vi "ActionVIOnDelete_RemoveSystemMappings.vi"(6 "All deleted Refs":T1[](array[typedef]) format="%.0x", 8 "error in (no error)":errorcluster, 11 "Item Ref in":T1 format="%.0x") -> (0 "error out":errorcluster, 3 "Item Ref out":T1 format="%.0x")   [LabVIEW 2015, in "Protection and Rolling Counter Addon System Explorer.lvlib"]
uses:
  Protection and Rolling Counter Addon System Explorer.lvlib
  <vilib>/NI Veristand/Custom Device API/Custom Device Item Ref.ctl
  Shared/Protection and Rolling Counter Addon Shared.lvlib
  <vilib>/NI Veristand/Custom Device API/Custom Device API.lvlib
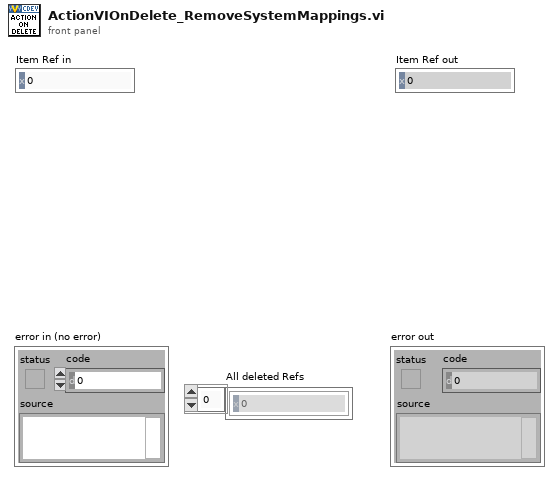
[diagram p1: front panel]
types:
  T1 = typedef "Custom Device API.lvlib/Custom Device Item Ref.ctl" = u64
  T2 = typedef "Protection and Rolling Counter Addon Shared.lvlib/FrameConfiguration.ctl" = cluster{"Input Channels":T3[], "Frame Rate":dbl, "Rolling Counter Count":dbl, "PCL Count":u64, "Max Count":dbl, "Frame ID":u32, "Rolling Counter":T3, "CRC":T3, "Frame Name":string, "Cluster":string, "Database":string, "Protection Type":T4}
  T3 = typedef "Protection and Rolling Counter Addon Shared.lvlib/InputChannelConfiguration.ctl" = cluster{"Start Bit":i32, "Name":string, "Node Path":string, "Number of bits":i32, "Scale":dbl, "Offset":dbl, "Data Type":u32}
  T4 = typedef "Protection and Rolling Counter Addon Shared.lvlib/Protection Type.ctl" = enum16{"Checksum", "CRC", "None (Counter Only)"}
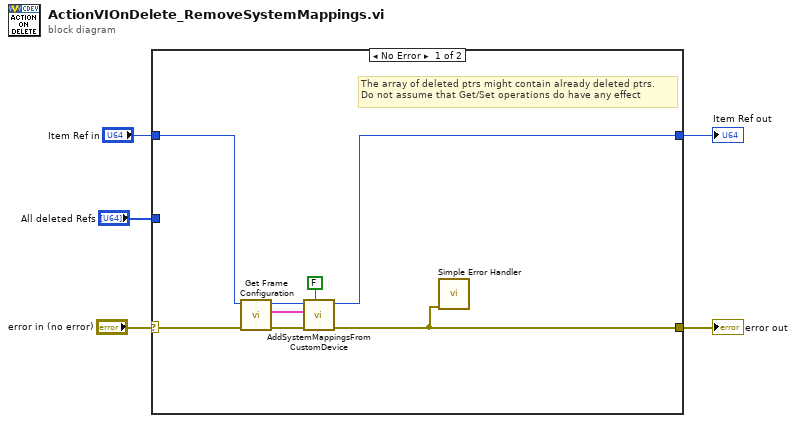
[diagram p0: block diagram]
diagram:
  n1 = case shown="No Error" "error in (no error)" {
    selector: "error in (no error)" -> [w12 w15]
    tunnel: [w6 w15] -> w4
    tunnel: "Item Ref in" -> [w11 w14]
    tunnel: [w8 w14] -> w2
    tunnel: "All deleted Refs" -> [_ _]
    frame No Error {
      # "The array of deleted ptrs might contain already deleted ptrs.\nDo not assume that Get/Set operations do have any effect"
      n2 = call "Get Frame Configuration.vi"("error in"=w12, "Parent Ref"=w11) -> ("error out"=w7:errorcluster, "Selected Channels"=w10:T2, "Parent Ref Out"=w9:T1)  [unwired: 7 in]
      n3 = call "AddSystemMappingsFromCustomDevice.vi"("Add? (T)"=FALSE, "error in"=w7, "Frame Configuration"=w10, "Node Ptr"=w9) -> ("error out"=w6:errorcluster, "Section Ref out"=w8:T1)  [unwired: 5 in, 1 out]
      n4 = call <vilib>:"Simple Error Handler.vi"("error in (no error)"=w6) -> ()  [unwired: 4 in, 5 out]
    }
    frame Error {
    }
  }
  "error out" <- w4
  "Item Ref out" <- w2
